vi "log printer sent msg.vi"(8 "error in (no error)":errorcluster, 11 "new element/subarray":string) -> (0 "error out":errorcluster, 3 "sent 2":string[](array[string]))   [LabVIEW 2015]
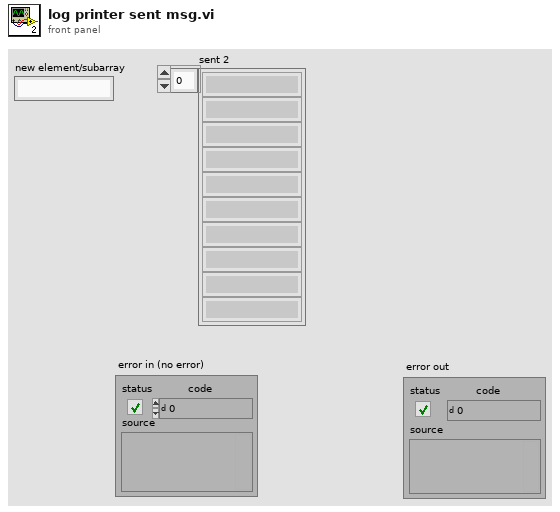
[diagram p1: front panel]
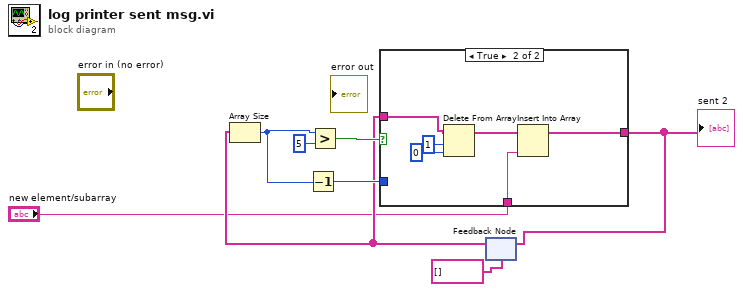
[diagram p0: block diagram]
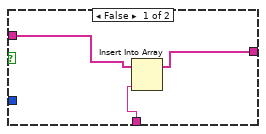
[diagram p2: hidden frame]
diagram:
  n1 = feedback #1(string[] [] ("sent 2")) -> (w3:string[])
  n2 = Array Size(array=w3) -> (size(s)=w6:i32)
  n3 = Decrement(x=w6) -> (x-1=w5:i32)
  n4 = Greater?(x=w6, y=5) -> (0:w7:bool)
  n5 = case shown="True" w7 {
    tunnel: w5 -> [_ _]
    tunnel: w3 -> [w11 w16]
    tunnel: [w9 w14] -> w4
    tunnel: "new element/subarray" -> [w10 w13]
    frame False {
      n6 = Insert Into Array(array=w11, new element=w10) -> (w9:string[])  [unwired: 1 in]
    }
    frame True {
      n7 = Delete From Array(array=w16, length=1, index=0) -> (array with subset deleted=w15:string[])  [unwired: 1 out]
      n8 = Insert Into Array(array=w15, new element=w13) -> (w14:string[])  [unwired: 1 in]
    }
  }
  "sent 2" <- w4
  n9 = feedback-in #1(w4) -> ()
